vi "5492_GearShake.vi"(8 "error in (no error)":errorcluster, 11 "RobotDriveDevRef":T1={"DevStatus"={"status"=FALSE, "code"=0, "source"=""}, "Motors[]"=[], "Square Inputs"=FALSE, "Max Output"=1.0}) -> (0 "error out (no error)":errorcluster, 3 "RobotDriveDevRef":T1={"DevStatus"={"status"=FALSE, "code"=0, "source"=""}, "Motors[]"=[], "Square Inputs"=FALSE, "Max Output"=1.0})   [LabVIEW 2016]
uses:
  <vilib>/Rock Robotics/WPI/RobotDrive/WPI_RobotDriveDevRef.ctl
  <vilib>/Rock Robotics/WPI/MotorControl/WPI_MotorControlDeviceRef.ctl
  <vilib>/Rock Robotics/WPI/MotorControl/WPI_MotorControlType.ctl
  <vilib>/Rock Robotics/SystemInterfaces/DIO/FPGA_DIOPWMChannel.ctl
  <vilib>/Rock Robotics/WPI/PWM/WPI_PWMDeadband.ctl
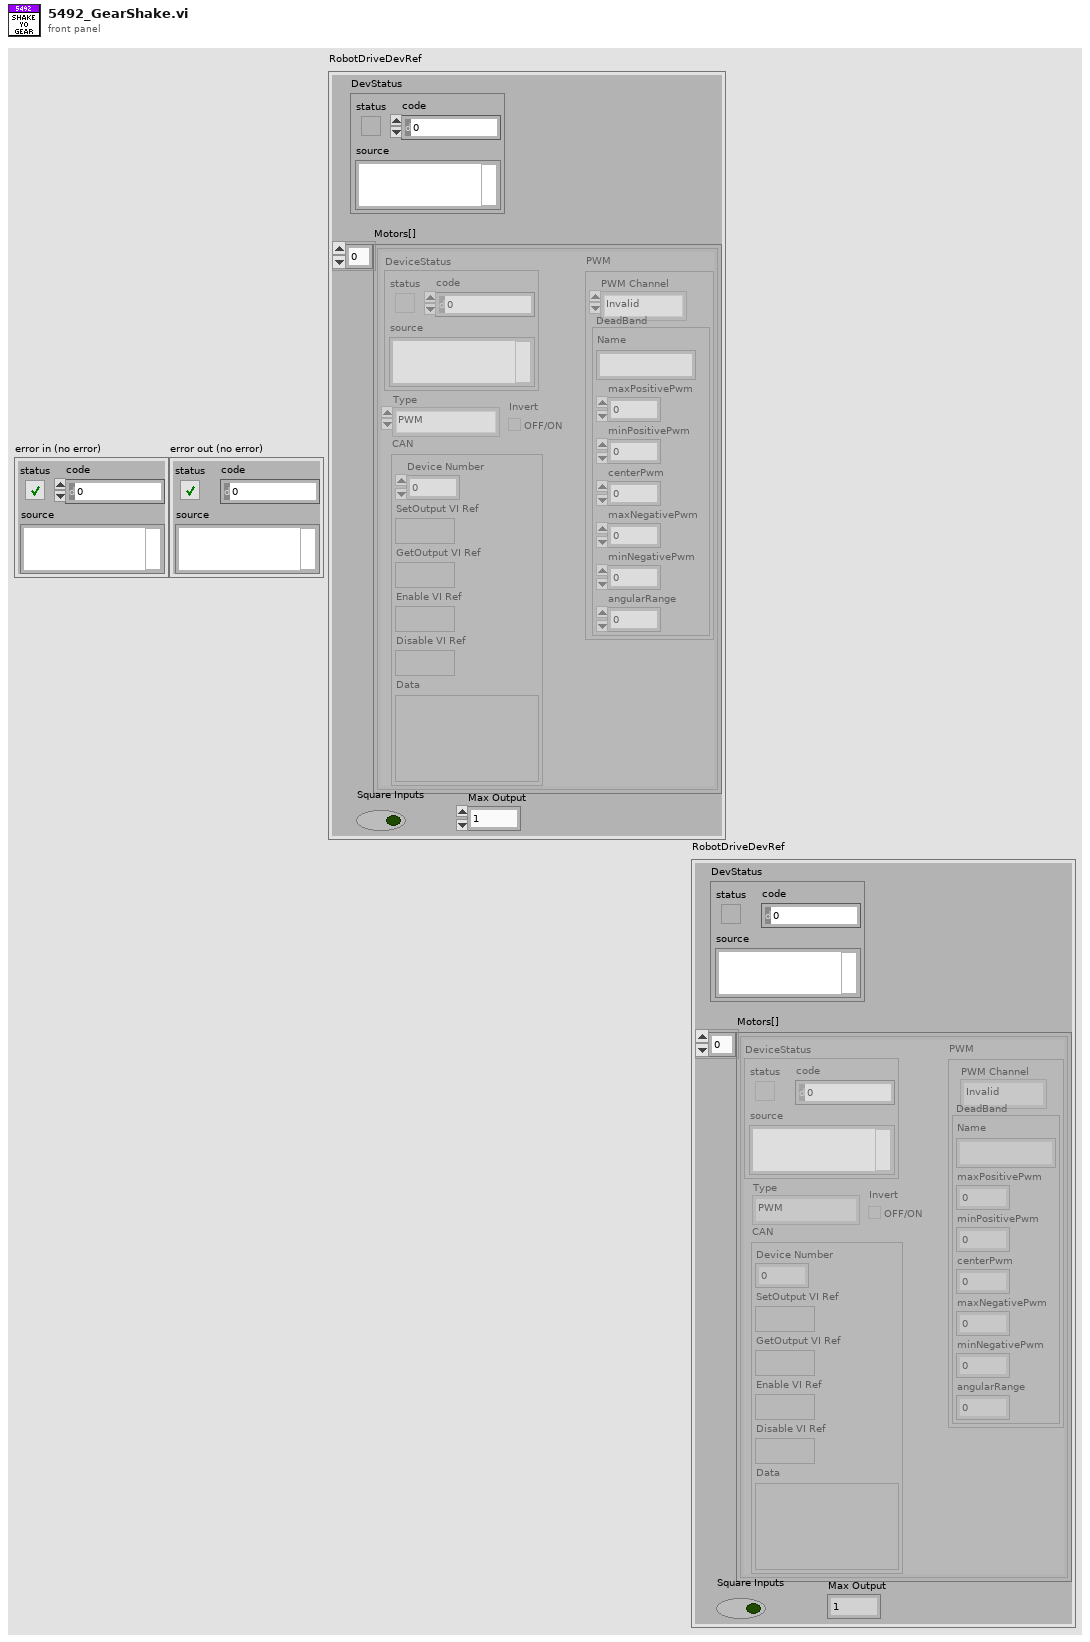
[diagram p1: front panel]
types:
  T1 = typedef "WPI_RobotDriveDevRef.ctl" = cluster{"DevStatus":errorcluster, "Motors[]":T2[], "Square Inputs":bool, "Max Output":dbl}
  T2 = typedef "WPI_MotorControlDeviceRef.ctl" = cluster{"DeviceStatus":errorcluster, "Type":T3, "PWM":cluster{"PWM Channel":T4, "DeadBand":T5}, "CAN":cluster{"Device Number":u8, "SetOutput VI Ref":variant, "GetOutput VI Ref":variant, "Enable VI Ref":variant, "Disable VI Ref":variant, "Data":variant}, "Invert":bool}
  T3 = typedef "WPI_MotorControlType.ctl" = enum16{"PWM", "CAN"}
  T4 = typedef "FPGA_DIOPWMChannel.ctl" = enum8{"PWM 0", "PWM 1", "PWM 2", "PWM 3", "PWM 4", "PWM 5", "PWM 6", "PWM 7", "PWM 8", "PWM 9", "PWM MXP 0", "PWM MXP 1", "PWM MXP 2", "PWM MXP 3", "PWM MXP 4", "PWM MXP 5", "PWM MXP 6", "PWM MXP 7", "PWM MXP 8", "PWM MXP 9", "Invalid"}
  T5 = typedef "WPI_PWMDeadband.ctl" = cluster{"Name":string, "maxPositivePwm":i32, "minPositivePwm":i32, "centerPwm":i32, "maxNegativePwm":i32, "minNegativePwm":i32, "angularRange":u16}
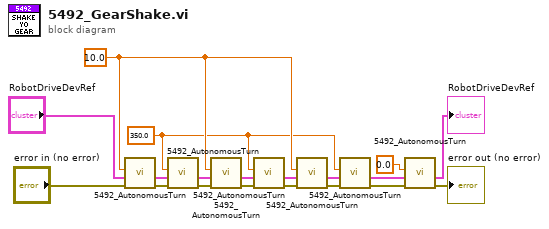
[diagram p0: block diagram]
diagram:
  w13 = 350.0
  w14 = 10.0
  n1 = call "5492_AutonomousTurn.vi"("error in (no error)"="error in (no error)", "RobotDriveDevRef"="RobotDriveDevRef", "Yaw Goallll"=w14) -> ("error out (no error)"=w7:errorcluster, "RobotDriveDevRef Output"=w19:T1)  [unwired: 7 in]
  n2 = call "5492_AutonomousTurn.vi"("error in (no error)"=w7, "RobotDriveDevRef"=w19, "Yaw Goallll"=w13) -> ("error out (no error)"=w6:errorcluster, "RobotDriveDevRef Output"=w18:T1)  [unwired: 7 in]
  n3 = call "5492_AutonomousTurn.vi"("error in (no error)"=w6, "RobotDriveDevRef"=w18, "Yaw Goallll"=w14) -> ("error out (no error)"=w5:errorcluster, "RobotDriveDevRef Output"=w17:T1)  [unwired: 7 in]
  n4 = call "5492_AutonomousTurn.vi"("error in (no error)"=w5, "RobotDriveDevRef"=w17, "Yaw Goallll"=w13) -> ("error out (no error)"=w4:errorcluster, "RobotDriveDevRef Output"=w16:T1)  [unwired: 7 in]
  n5 = call "5492_AutonomousTurn.vi"("error in (no error)"=w4, "RobotDriveDevRef"=w16, "Yaw Goallll"=w14) -> ("error out (no error)"=w3:errorcluster, "RobotDriveDevRef Output"=w15:T1)  [unwired: 7 in]
  n6 = call "5492_AutonomousTurn.vi"("error in (no error)"=w3, "RobotDriveDevRef"=w15, "Yaw Goallll"=w13) -> ("error out (no error)"=w2:errorcluster, "RobotDriveDevRef Output"=w12:T1)  [unwired: 7 in]
  n7 = call "5492_AutonomousTurn.vi"("error in (no error)"=w2, "RobotDriveDevRef"=w12, "Yaw Goallll"=0.0) -> ("error out (no error)"=→"error out (no error)":errorcluster, "RobotDriveDevRef Output"=→"RobotDriveDevRef":T1)  [unwired: 7 in]
